vi "Read User Project Path.vi"(8 "error in":errorcluster, 11 "PluginGenerator_MetaDataObj in":refnum<class "PluginGenerator_MetaDataObj.lvclass">) -> (0 "error out":errorcluster, 2 "User Project Path":path, 3 "PluginGenerator_MetaDataObj out":refnum<class "PluginGenerator_MetaDataObj.lvclass">)   [LabVIEW 2023, in "Plugin Generator.lvlib" / "PluginGenerator_MetaDataObj.lvclass"]
uses:
  PluginGenerator_MetaDataObj.lvclass
  c:/perforce/build/exports/ni/nito/nitoolchainlabview2023eng64/official/export/23.3/23.3.0f52/win/resource/dialog/NewProjectWizard/MetaDataObj/MetaDataObj.lvclass
  <resource>/dialog/NewProjectWizard/MetaDataObj/MetaDataObj.lvclass/MetaDataObj.ctl
  <resource>/dialog/NewProjectWizard/MetaDataObj/Accessors/Read Project Root.vi
  <resource>/dialog/NewProjectWizard/MetaDataObj/Accessors/Read Project Name.vi
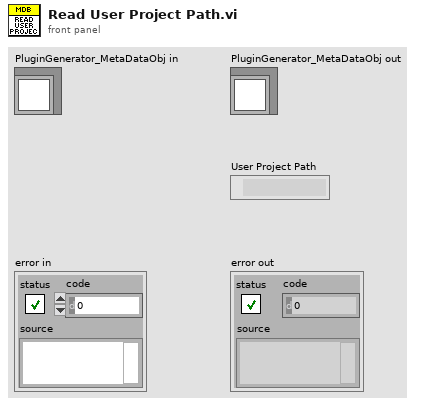
[diagram p1: front panel]
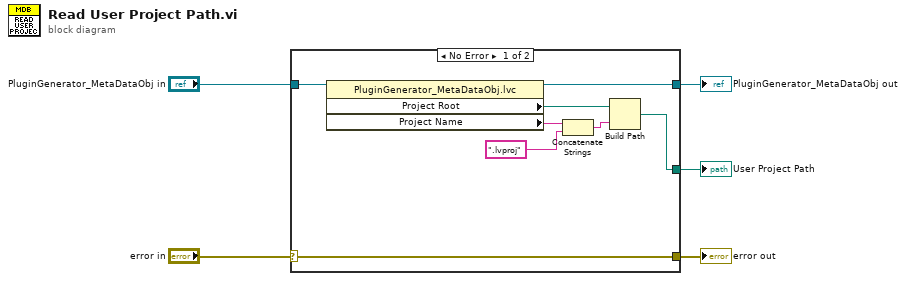
[diagram p0: block diagram]
diagram:
  n1 = case shown="No Error" "error in" {
    selector: "error in" -> [w13 w14]
    tunnel: [w13 w14] -> w4
    tunnel: [w6 w15] -> w2
    tunnel: "PluginGenerator_MetaDataObj in" -> [w12 w15]
    tunnel: [w7 _] -> w1
    frame No Error {
      n2 = property class="PluginGenerator_MetaDataObj.lvc"(reference=w12) -> (reference out=w6:refnum<class "PluginGenerator_MetaDataObj.lvclass">, "Project Root"=w8:path, "Project Name"=w11:string)  [unwired: 1 in, 1 out]
      n3 = Concatenate Strings(w11, ".lvproj" ("string")) -> (w9:string)
      n4 = Build Path(base path=w8, name or relative path=w9) -> (appended path=w7:path)
    }
    frame Error {
    }
  }
  "error out" <- w4
  "PluginGenerator_MetaDataObj out" <- w2
  "User Project Path" <- w1
